vi "unregisterPublisher.vi"(1 "Parameters":T3) -> (2 "Error out":errorcluster, 3 "Reply":T2, 4 "Log":T1)   [LabVIEW 2010]
uses:
  _ROSDefinition.vi
  Console/Servers/ServerSubs/ROSLog.ctl
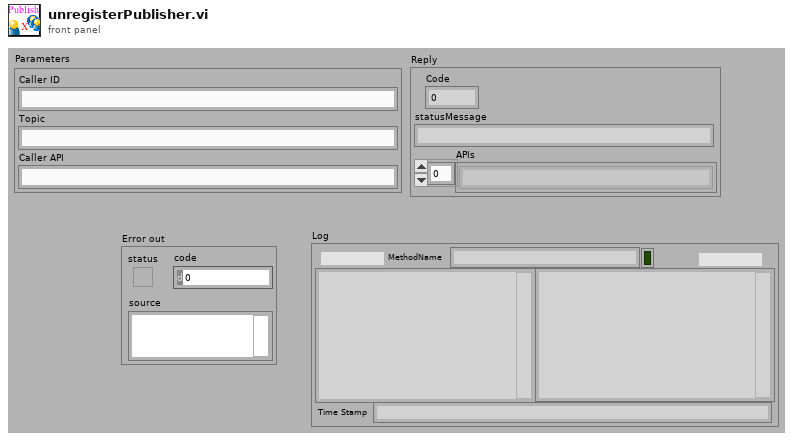
[diagram p1: front panel]
types:
  T1 = typedef "ROSLog.ctl" = cluster{"Sent":string, "Reply":string, "MethodName":string, "success":bool, "Dir1":string, "Dir2":string, "Time Stamp":string}
  T2 = cluster{"Code":i8, "statusMessage":string, "APIs":string[]}
  T3 = cluster{"Caller ID":string, "Topic":string, "Caller API":string}
  T4 = cluster{"Code":i8, "statusMessage":string, "APIs":string[]}[]
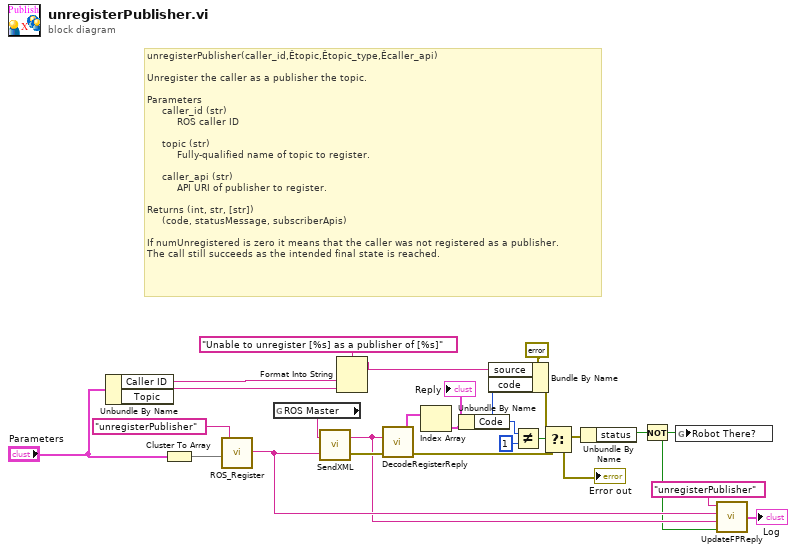
[diagram p0: block diagram]
diagram:
  # "unregisterPublisher(caller_id,Êtopic,Êtopic_type,Êcaller_api)\n\nUnregister the caller as a publisher the topic. \n\nParameters \n     caller_id (str) \n          ROS caller ID\n\n     topic (str) \n          Fully-qualified name of topic to register.\n\n     caller_api (str) \n          API URI of publisher to register.\n\nReturns (int, str, [str]) \n     (code, statusMessage, subscriberApis) \n\nIf numUnregistered is zero it means that the caller was not registered as a publisher. \nThe call still succeeds as the intended final state is reached."
  n1 = Unbundle By Name("Parameters") -> ("Caller ID"=w21:string, "Topic"=w20:string)
  n2 = Cluster To Array(cluster="Parameters") -> (array=w6:string[])
  n3 = call "ROS_Register.vi"("Parameters"=w6, "Method Name"="unregisterPublisher") -> ("registerSubscriber"=w4:string)  [unwired: 1 in]
  n4 = global read "_ROSDefinition.vi" "ROS Master"() -> (w24:string)
  n5 = call "SendXML.vi"("Send"=w4, "URI in"=w24) -> ("error out"=w10:errorcluster, "Reply"=w3:string)
  n6 = Format Into String(format string="Unable to unregister [%s] as a publisher of [%s]" ("source"), w21, w20) -> (resulting string=w9:string)  [unwired: 2 in, 1 out]
  n7 = call "DecodeRegisterReply.vi"("error in (no error)"=w10, "Response"=w3) -> ("error out"=w14:errorcluster, "Reply"=w18:T4)
  n8 = Index Array(array=w18) -> (element=w17:T2)  [unwired: 1 in]
  "Reply" <- w17
  n9 = Unbundle By Name(w17) -> ("Code"=w13:i8)
  n10 = Bundle By Name(cluster=errorcluster {"status"=TRUE, "code"=0, "source"=" Error"} ("t"), "source"=w9, "code"=w13) -> (w12:errorcluster)
  n11 = Not Equal?(x=w13, y=i8 1) -> (x != y?=w15:bool)
  n12 = Select(t=w12, s=w15, f=w14) -> (s? t:f=w11:errorcluster)
  "Error out" <- w11
  n13 = Unbundle By Name(w11) -> ("status"=w19:bool)
  n14 = Not(x=w19) -> (.not. x?=w2:bool)
  n15 = global write "_ROSDefinition.vi" "Robot There?"(w2) -> ()
  n16 = call "UpdateFPReply.vi"("success?"=w2, "Reply"=w3, "Sent"=w4, "method"="unregisterPublisher" ("name (unnamed)")) -> ("Log"=→"Log":T1)
